vi "Init Module.vi"(8 "error in (no error)":errorcluster, 11 "TestModule in":refnum<class "TestModule.lvclass">) -> (0 "error out":errorcluster, 3 "TestModule out":refnum<class "TestModule.lvclass">)   [LabVIEW 2020, in "VolatusScratch.lvlib" / "TestModule.lvclass"]
uses:
  TestModule.lvclass
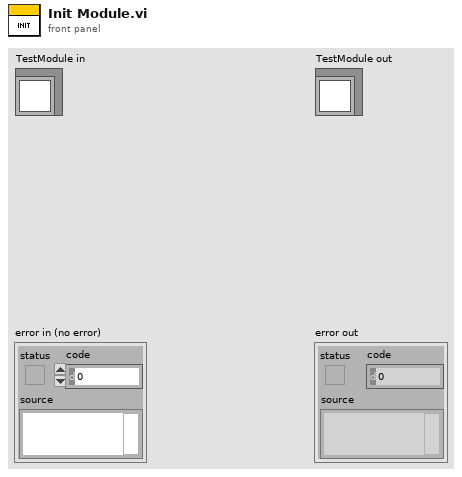
[diagram p1: front panel]
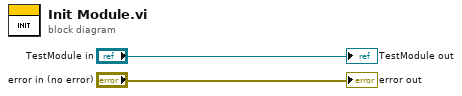
[diagram p0: block diagram]
diagram:
  "error out" <- "error in (no error)"
  "TestModule out" <- "TestModule in"
